vi "GetRunModes.vi"(8 "Error In":errorcluster, 11 "Item Symbols In":i32[](array[numeric])) -> (0 "Error Out":errorcluster, 3 "Run Modes Out":string[](array[string]))   [LabVIEW 2011]
doc: "This VI will convert ItemSymbols Array to String Array."
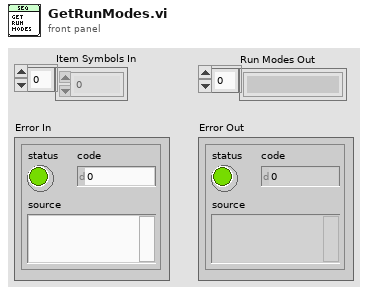
[diagram p1: front panel]
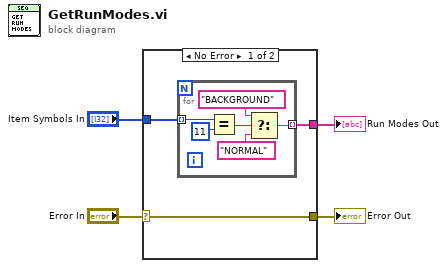
[diagram p0: block diagram]
diagram:
  n1 = case shown="No Error" "Error In" {
    selector: "Error In" -> [w5 w14]
    tunnel: "Item Symbols In" -> [w7 _]
    tunnel: [w6 _] -> w3
    tunnel: [w5 w14] -> w1
    frame No Error {
      n2 = for {
        tunnel: w7 -> [w13] mode=indexing
        tunnel: [w8] -> w6 mode=indexing
        n3 = Equal?(x=w13, y=11) -> (x = y?=w11:bool)
        n4 = Select(t="BACKGROUND" ("Queue Name In"), s=w11, f="NORMAL" ("Queue Name In")) -> (s? t:f=w8:string)
      }
    }
    frame Error {
    }
  }
  "Run Modes Out" <- w3
  "Error Out" <- w1
